vi "Get Element Changed Event.vi"(8 "error in (no error)":errorcluster, 11 "ControlArray in":refnum<class "ControlArray.lvclass">) -> (0 "error out":errorcluster, 2 "Element Changed":refnum<user-event>, 3 "ControlArray out":refnum<class "ControlArray.lvclass">)   [LabVIEW 2020, in "Control Array.lvlib" / "ControlArray.lvclass"]
uses:
  ControlArray.lvclass
  Element Changed Event Data.ctl
  ControlArray.lvclass/ControlArray.ctl
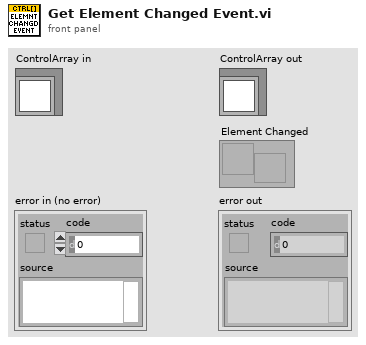
[diagram p1: front panel]
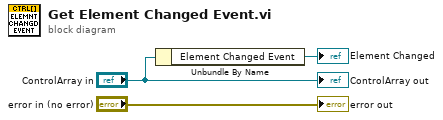
[diagram p0: block diagram]
diagram:
  n1 = Unbundle By Name("ControlArray in") -> ("Element Changed Event"=→"Element Changed":refnum<user-event>)
  "error out" <- "error in (no error)"
  "ControlArray out" <- "ControlArray in"
